vi "Capture@ClearImaq__Parameter.vi"(1 "ParamterIn":string) -> (0 "ParamterOut":string)   [LabVIEW 2020]
panel:
  in  "IMAQName":string(combo)
  in  "Confirm":bool
  # "Capture@Snap $ImaqName"
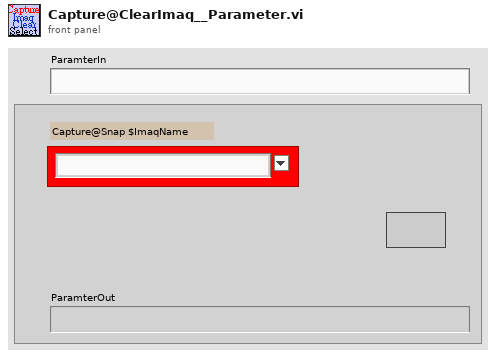
[diagram p1: front panel]
types:
  T1 = enum16{"Get", "Get&Index+1", "Insert", "Init", "Clear", "SetIndex"}
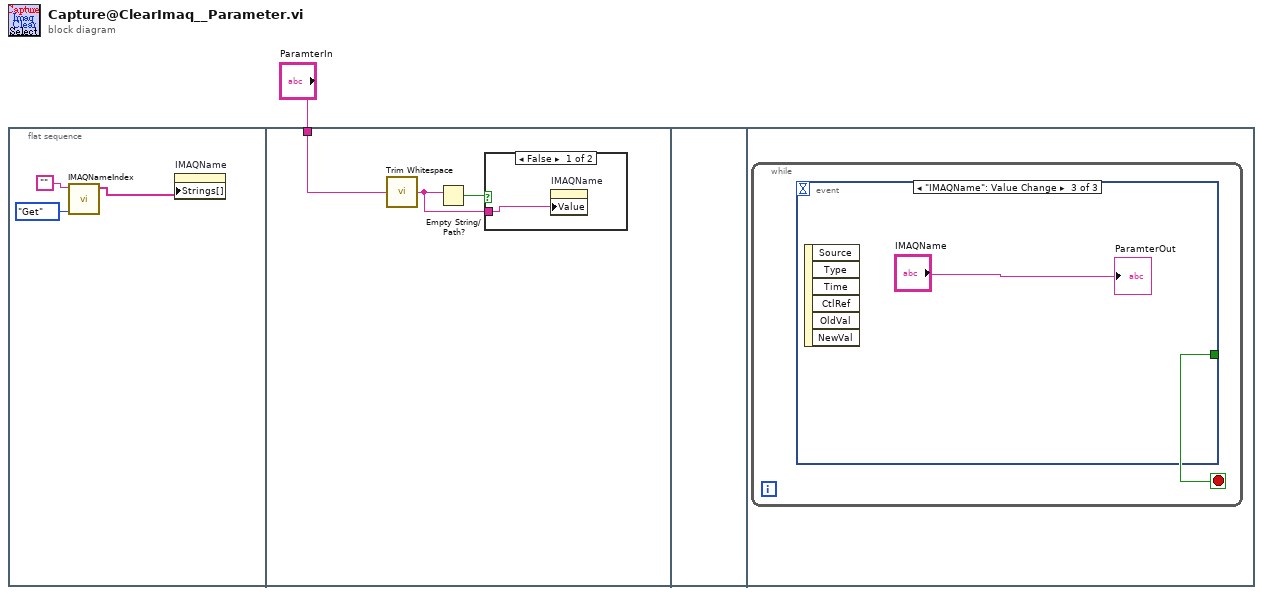
[diagram p0: block diagram]
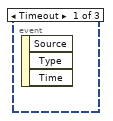
[diagram p3: hidden frame]
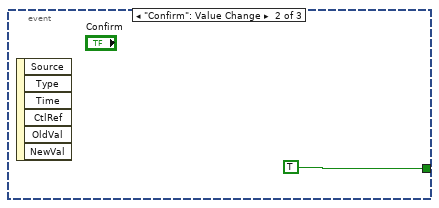
[diagram p4: hidden frame]
diagram:
  n1 = flat-sequence {
    tunnel: "ParamterIn" -> [w5]
    frame #0 {
      n2 = call "IMAQNameIndex.vi"("OP"=T1."Get", "IMAQName"="") -> ("IMAQNameList"=w2:string[])  [unwired: 2 in, 7 out]
      n3 = property on="IMAQName" class="CmbBox"("Strings[]"=w2) -> ()  [unwired: 2 in, 2 out]
    }
    frame #1 {
      n4 = call <vilib>:"Trim Whitespace.vi"("string"=w5) -> ("trimmed string"=w6:string)  [unwired: 1 in]
      n5 = Empty String/Path?(string/path=w6) -> (empty?=w7:bool)
      n6 = case shown="False" w7 {
        tunnel: w6 -> [w8 _]
        frame False {
          n7 = property on="IMAQName" class="CmbBox"("Value"=w8) -> ()  [unwired: 2 in, 2 out]
        }
        frame True {
        }
      }
    }
    frame #2 {
    }
    frame #3 {
      n8 = while {
        stop <- w9 stop-if-true
        n9 = event shown="[2] \"IMAQName\": Value Change" {
          selector: _ -> [_ _ _]
          dyn-events: _ -> [_ _ _]
          timeout: _ -> [_ _ _]
          tunnel: [_ TRUE _] -> w9
          event Timeout {
            n10 = event-data() -> ()  [unwired: 1 in, 3 out]
          }
          event "Confirm": Value Change {
            n11 = event-data() -> ()  [unwired: 1 in, 6 out]
          }
          event "IMAQName": Value Change {
            n12 = event-data() -> ()  [unwired: 1 in, 6 out]
            "ParamterOut" <- "IMAQName"
          }
        }
      }
    }
  }
